vi "Note Popup Setup.vi"(6 "SR Number":i32, 8 "error in":errorcluster, 9 "Main VI ref in":refnum<vi>, 10 "This VI in":refnum<vi>, 11 "string ref in":refnum<vi>) -> (0 "error out":errorcluster, 1 "Main VI ref out":refnum<vi>, 2 "This VI out":refnum<vi>, 3 "string ref out":refnum<vi>)   [LabVIEW 2018]
uses:
  <vilib>/Utility/miscctls.llb/LVPositionTypeDef.ctl
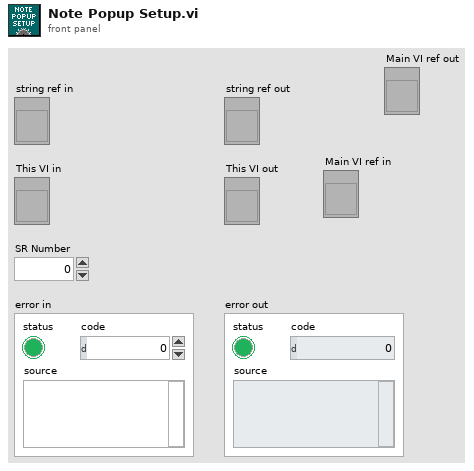
[diagram p1: front panel]
types:
  T1 = typedef "LVPositionTypeDef.ctl" = cluster{"Left":i32, "Top":i32}
  T2 = enum16{"Always On", "Always Off", "Off While Running"}
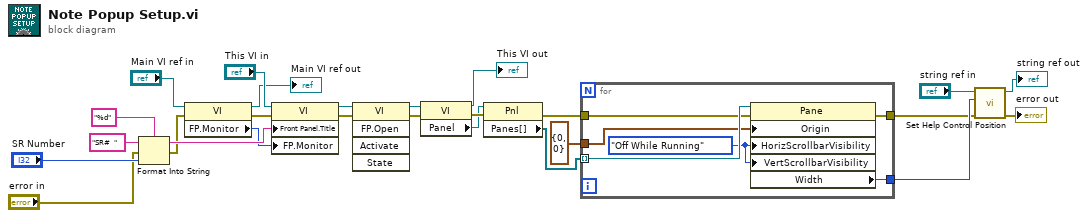
[diagram p0: block diagram]
diagram:
  n1 = Format Into String(format string="%d", initial string="SR#  ", error in="error in", "SR Number") -> (resulting string=w9:string, error out=w3:errorcluster)
  n2 = property class="VI"(reference="Main VI ref in", error in=w3) -> (reference out=→"Main VI ref out":refnum<vi>, error out=w5:errorcluster, "FP.Monitor"=w4:u16)
  n3 = property class="VI"(reference="This VI in", error in=w5, "Front Panel.Title"=w9, "FP.Monitor"=w4) -> (reference out=w20:refnum<vi>, error out=w21:errorcluster)
  n4 = invoke class="VI" method="FP.Open"(reference=w20, error in=w21) -> (reference out=w23:refnum<vi>, error out=w22:errorcluster)  [unwired: 3 in, 3 out]
  n5 = property class="VI"(reference=w23, error in=w22) -> (reference out=→"This VI out":refnum<vi>, error out=w25:errorcluster, "Panel"=w24:refnum<vi>)
  n6 = property class="Pnl"(reference=w24, error in=w25) -> (error out=w12:errorcluster, "Panes[]"=w13:refnum<vi>[])  [unwired: 1 out]
  n7 = for {
    tunnel: w13 -> [w32] mode=indexing
    tunnel: T1 {"Left"=0, "Top"=0} ("Position") -> [w31]
    tunnel: w12 -> [w30]
    tunnel: [w29] -> w15
    tunnel: [w27] -> w16
    w28 = T2."Off While Running" ("Horizontal Scrollbar Visibility")
    n8 = property class="Pane"(reference=w32, error in=w30, "Origin"=w31, "HorizScrollbarVisibility"=w28, "VertScrollbarVisibility"=w28) -> (error out=w29:errorcluster, "Width"=w27:u32)  [unwired: 1 out]
  }
  n9 = call "Set Help Control Position.vi"("error in (no error)"=w15, "Width"=w16, "String in"="string ref in") -> ("error out"=→"error out":errorcluster, "String out"=→"string ref out":refnum<vi>)  [unwired: 7 in]
